vi "niRFUtil MT UTIL Get Polyphase Filter.vi"(10 "# of zero crossings":i32=8, 11 "interpolation factor in":i32=512) -> (0 "effective filter length":i32=16, 1 "interpolation factor":i32=128, 2 "differencesBetweenCoeffs[]":T1 min=0 max=127 format="%.2f", 3 "scaledFilterCoefficients[]":T1 min=0 max=127 format="%.2f")   [LabVIEW 2015, in "niRFUtil.lvlib"]
uses:
  niRFUtil.lvlib
  Includes/niRFUtil INC Real Array.ctl
  niRFAMT.dll
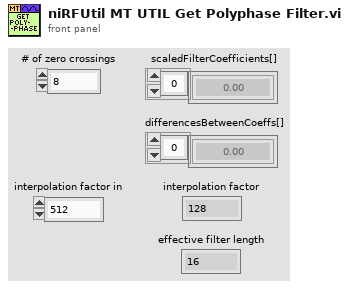
[diagram p1: front panel]
types:
  T1 = typedef "niRFUtil.lvlib/niRFUtil INC Real Array.ctl" = sgl[]
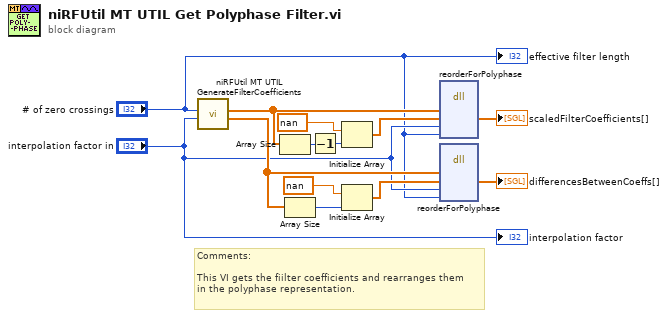
[diagram p0: block diagram]
diagram:
  # "Comments:\n\nThis VI gets the fiilter coefficients and rearranges them\nin the polyphase representation."
  n1 = call "niRFUtil MT UTIL GenerateFilterCoefficients.vi"("interpolation factor"="interpolation factor in", "# of zero crossings"="# of zero crossings") -> ("Differences (scaled)"=w5:T1, "Filter Coefficients (scaled)"=w12:T1)  [unwired: 1 in, 7 out]
  n2 = Array Size(array=w12) -> (size(s)=w13:i32)
  n3 = Array Size(array=w5) -> (size(s)=w10:i32)
  n4 = Decrement(x=w13) -> (x-1=w1:i32)
  n5 = Initialize Array(sgl nan ("element"), w1) -> (w11:sgl[])
  n6 = Initialize Array(sgl nan ("element"), w10) -> (w4:sgl[])
  n7 = dll-call lib="C:/Perforce/semoore-sales/Customers/NATI-3813/Noise Floor/LV Filters/ParallelComplexFilterRFUtil/niRFUtil/MT/Utilities/niRFAMT.*" fn="reorderForPolyphase"("arrayIn"=w12, "arrayOut"=w11, "interpolation factor"="interpolation factor in", "effective filter length"="# of zero crossings") -> ("arrayOut"=→"scaledFilterCoefficients[]":dbl[])  [unwired: 6 in, 3 out]
  n8 = dll-call lib="C:/Perforce/semoore-sales/Customers/NATI-3813/Noise Floor/LV Filters/ParallelComplexFilterRFUtil/niRFUtil/MT/Utilities/niRFAMT.*" fn="reorderForPolyphase"("arrayIn"=w5, "arrayOut"=w4, "interpolation factor"="interpolation factor in", "effective filter length"="# of zero crossings") -> ("arrayOut"=→"differencesBetweenCoeffs[]":dbl[])  [unwired: 6 in, 3 out]
  "interpolation factor" <- "interpolation factor in"
  "effective filter length" <- "# of zero crossings"
